vi "CustomDigMdGetDIO.vi"(8 "error in (no error)":errorcluster, 10 "DIOChannel":T3=enum."DIO 1", 11 "DigitalModuleDevRef 2":T1) -> (0 "error out":errorcluster, 2 "x .and. y?":u32, 3 "DigitalModuleDevRef":T1)   [LabVIEW 2014]
uses:
  <vilib>/Rock Robotics/SystemInterfaces/DIO/FPGA_DIOChannel.ctl
  <vilib>/Rock Robotics/WPI/DigitalModule/WPI_DigitalModuleDeviceRef.ctl
  <vilib>/Rock Robotics/SystemInterfaces/Typedef/FPGA_TypedefDigitalModule.ctl
  <vilib>/Rock Robotics/SystemInterfaces/System/FPGA_SystemGet.vi
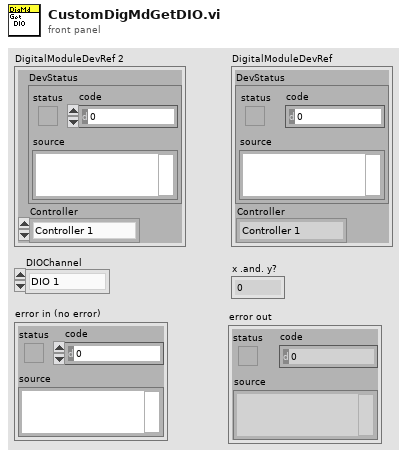
[diagram p1: front panel]
types:
  T1 = typedef "WPI_DigitalModuleDeviceRef.ctl" = cluster{"DevStatus":errorcluster, "Controller":T2}
  T2 = typedef "FPGA_TypedefDigitalModule.ctl" = enum16{"Controller 1"}
  T3 = typedef "FPGA_DIOChannel.ctl" = enum8{"DIO 0", "DIO 1", "DIO 2", "DIO 3", "DIO 4", "DIO 5", "DIO 6", "DIO 7", "DIO 8", "DIO 9", "DIO MXP 0", "DIO MXP 1", "DIO MXP 2", "DIO MXP 3", "DIO MXP 4", "DIO MXP 5", "DIO MXP 6", "DIO MXP 7", "DIO MXP 8", "DIO MXP 9", "DIO MXP 10", "DIO MXP 11", "DIO MXP 12", "DIO MXP 13", "DIO MXP 14", "DIO MXP 15", "Invalid"}
  T4 = typedef "FPGA_DIODevRef.ctl" = cluster{"DevStatus":errorcluster, "Controller":T2}
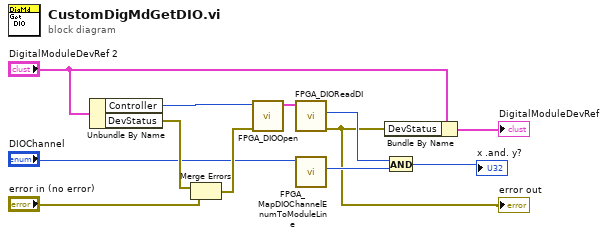
[diagram p0: block diagram]
diagram:
  n1 = Unbundle By Name("DigitalModuleDevRef 2") -> ("Controller"=w10:T2, "DevStatus"=w11:errorcluster)
  n2 = Merge Errors(w11, "error in (no error)") -> (w12:errorcluster)
  n3 = call <vilib>:"FPGA_DIOOpen.vi"("error in (no error)"=w12, "Controller"=w10) -> ("DIODeviceRef"=w7:T4)  [unwired: 9 out]
  n4 = call <vilib>:"FPGA_DIOReadDI.vi"("DIODeviceRef In"=w7) -> ("error out"=w3:errorcluster, "DI"=w8:u32)  [unwired: 1 in, 8 out]
  "error out" <- w3
  n5 = call <vilib>:"FPGA_MapDIOChannelEnumToModuleLine.vi"("DIOChannel"="DIOChannel") -> ("ActualDIOBitMask(U32)"=w9:u32)  [unwired: 10 out]
  n6 = Bundle By Name(cluster="DigitalModuleDevRef 2", "DevStatus"=w3) -> (→"DigitalModuleDevRef":T1)
  n7 = And(x=w8, y=w9) -> (x .and. y?=→"x .and. y?":u32)
